vi "TCP HeartBeat Generator.vi"() -> ()   [LabVIEW 2018]
panel:
  out "HeartBeat Array Size":i32
  in  "HeartBeat Period (s)":dbl=4.0 format="%#_13g"
  out "HeartBeat Array":string[](array[string])
  out "bytes written":i32
  in  "HeartBeat Content":string="HeartBeatMessage"
  in  "error in (no error)":errorcluster
  out "error out":errorcluster
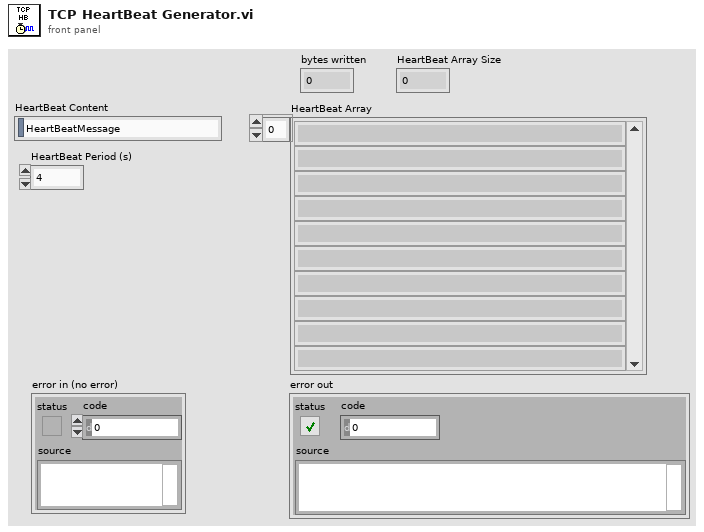
[diagram p1: front panel]
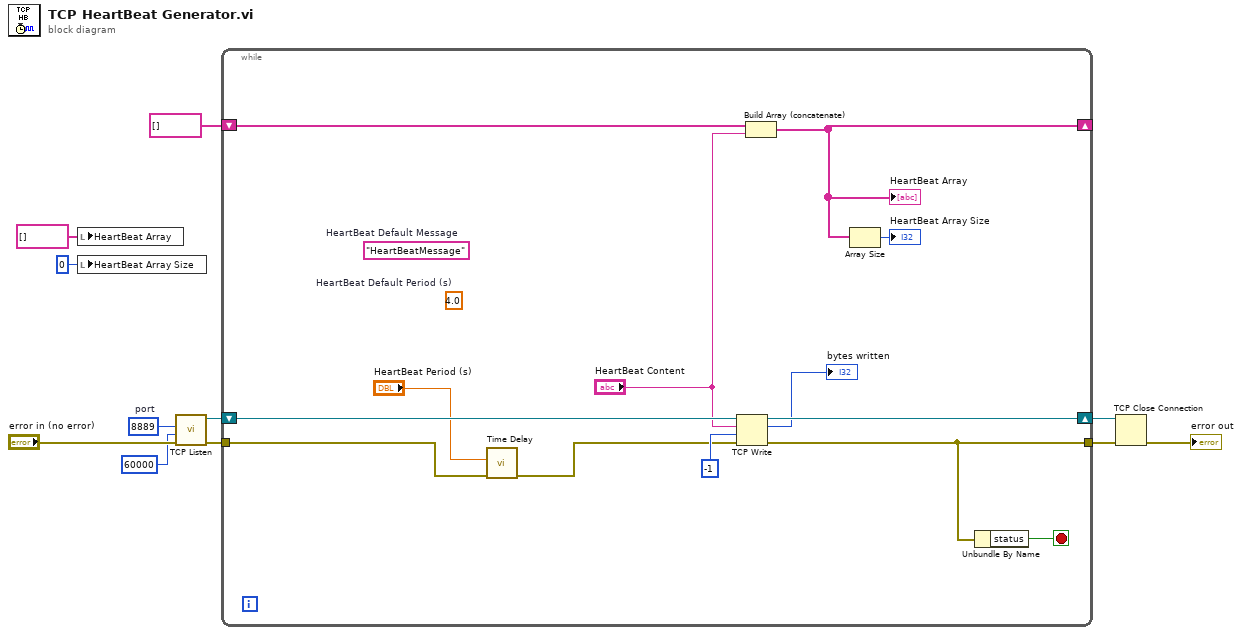
[diagram p0: block diagram]
diagram:
  w8 = u16 8889  # port
  n1 = local write "HeartBeat Array"(string[] [] ("HeartBeat Array")) -> ()
  n2 = local write "HeartBeat Array Size"(0 ("HeartBeat Array Size")) -> ()
  n3 = call <vilib>:"TCP Listen.vi"("error in (no error)"="error in (no error)", "timeout ms (wait forever: -1)"=60000, "port"=w8) -> ("error out"=w6:errorcluster, "connection ID"=w7:refnum<k5>)  [unwired: 4 in, 3 out]
  n4 = while {
    shift-right: [w13] -> _
    shift-left: string[] [] -> [w23]
    shift-right: [w20] -> w11
    shift-left: w7 -> [w24]
    tunnel: w6 -> [w14]
    tunnel: [w21] -> w10
    stop <- w22 stop-if-true
    (unwired) 4.0  # HeartBeat Default Period (s)
    (unwired) "HeartBeatMessage"  # HeartBeat Default Message
    n5 = call "Time Delay"("error in (no error)"=w14, "Delay Time (s)"="HeartBeat Period (s)") -> ("error out"=w15:errorcluster)  [unwired: 9 in]
    n6 = TCP Write(connection ID=w24, data in="HeartBeat Content", error in (no error)=w15, 9:-1 ("timeout ms (25000)")) -> (connection ID out=w20:refnum<k5>, bytes written=→"bytes written":i32, error out=w21:errorcluster)
    n7 = Build Array (concatenate)(w23, "HeartBeat Content") -> (w13:string[])
    "HeartBeat Array" <- w13
    n8 = Array Size(array=w13) -> (size(s)=→"HeartBeat Array Size":i32)
    n9 = Unbundle By Name(w21) -> ("status"=w22:bool)
  }
  n10 = TCP Close Connection(connection ID=w11, error in (no error)=w10) -> (error out=→"error out":errorcluster)  [unwired: 1 in, 1 out]
